vi "Configure Constant Resistance.vi"(8 "error in (no error)":errorcluster, 10 "CR Resistance (1)":dbl=1.0 min=0.05 max=7500.0 step=1.0 format="%#.4g", 11 "VISA resource name":refnum<visa-resource-name>) -> (0 "error out":errorcluster, 3 "VISA resource name out":refnum<visa-resource-name>)   [LabVIEW 2024, in "BK Precision 8500B Series.lvlib"]
doc: "Configures the resistance for constant resistance (CR) operation."
uses:
  BK Precision 8500B Series.lvlib
panel:
  # "Ohm"
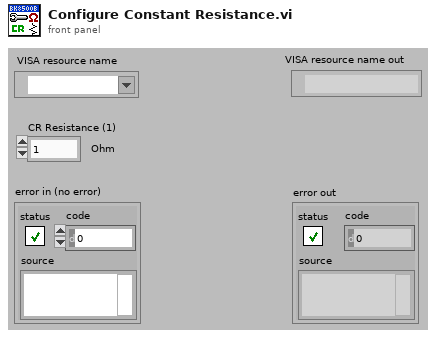
[diagram p1: front panel]
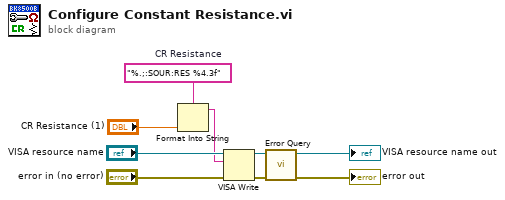
[diagram p0: block diagram]
diagram:
  w7 = "%.;:SOUR:RES %4.3f"  # CR Resistance
  n1 = Format Into String(format string=w7, "CR Resistance (1)") -> (resulting string=w1:string)  [unwired: 2 in, 1 out]
  n2 = VISA Write(VISA resource name="VISA resource name", write buffer=w1, error in (no error)="error in (no error)") -> (VISA resource name out=w5:refnum<visa-resource-name>, error out=w6:errorcluster)  [unwired: 1 out]
  n3 = call "Error Query.vi"("error in (no error)"=w6, "VISA resource name"=w5) -> ("error out"=→"error out":errorcluster, "VISA resource name out"=→"VISA resource name out":refnum<visa-resource-name>)  [unwired: 6 in, 2 out]
